vi "Stop.vi"(8 "error in (no error)":errorcluster, 11 "Sequence in":refnum<class "Sequence.lvclass">) -> (0 "error out":errorcluster, 3 "Sequence out":refnum<class "Sequence.lvclass">)   [LabVIEW 2018, in "Sequence.lvclass"]
doc: "Advance\ncounter to STOP\nthen continue\nwithin the \nSequence case"
uses:
  Sequence.lvclass
  Sequence.lvclass/Sequence.ctl
  SequenceSubvis/TestStepTypes.ctl
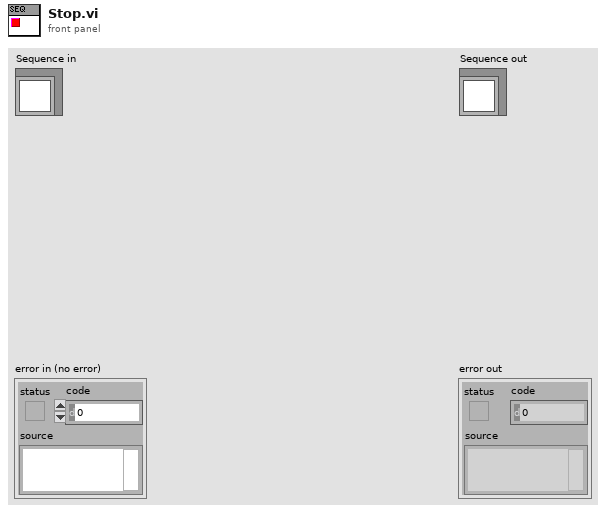
[diagram p1: front panel]
types:
  T1 = typedef "TestStepTypes.ctl" = enum16{"MotionFF-M2", "Motion", "SweepTest", "RasterTest", "Finish", "64ModuleCfg"}
  T2 = typedef "mWaveTestStep.ctl" = cluster{"StepType":T1, "RF In/Out":T3, "Module/Raster":i32, "Polarization":T4, "AO-64 Array":dbl[], "Position":T5[]}
  T3 = typedef "RF Direction.ctl" = enum16{"Tx - RF In", "Rx - RF Out"}
  T4 = typedef "PolarizationSelect.ctl" = enum16{"Vertical", "Horizontal"}
  T5 = typedef "singleAxisMoveDef.ctl" = cluster{"mmWave Axis":T6, "eng. value":dbl}
  T6 = typedef "mmWaveAxis.ctl" = string
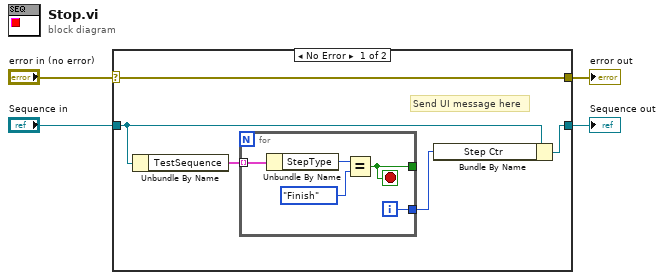
[diagram p0: block diagram]
diagram:
  n1 = case shown="No Error" "error in (no error)" {
    selector: "error in (no error)" -> [w9 w16]
    tunnel: [w9 w16] -> w3
    tunnel: [w6 w15] -> w1
    tunnel: "Sequence in" -> [w7 w15]
    frame No Error {
      # "Send UI message here"
      n2 = Unbundle By Name(w7) -> ("TestSequence"=w8:T2[])
      n3 = for {
        tunnel: w8 -> [w14] mode=indexing
        tunnel: [w13] -> _
        tunnel: [w12] -> w5
        i -> [w12]
        stop <- w13 stop-if-true
        n4 = Unbundle By Name(w14) -> ("StepType"=w11:T1)
        n5 = Equal?(x=w11, y=TestStepTypes."Finish" ("StepType")) -> (x = y?=w13:bool)
      }
      n6 = Bundle By Name(cluster=w7, "Step Ctr"=w5) -> (w6:refnum<class "Sequence.lvclass">)
    }
    frame Error {
    }
  }
  "error out" <- w3
  "Sequence out" <- w1
